vi "Dales Analog Read Pin.vi"(0 "Arduino Resource":T1={"VISA resource"="COM11", "Board Type"=enum."Uno", "Connection Type"=enum."USB / Serial", "Bytes Per Packet (15)"=15}, 7 "Analog Input Pin (0)":u8, 11 "error in":errorcluster) -> (4 "Arduino Resource":T1={"VISA resource"="COM11", "Board Type"=enum."Uno", "Connection Type"=enum."USB / Serial", "Bytes Per Packet (15)"=15}, 15 "error out":errorcluster)   [LabVIEW 2010]
doc: "Reads the analog voltage on the selected Arduino analog input pin (A0 - A5)."
uses:
  <vilib>/LabVIEW Interface for Arduino/Type Defs/Arduino Resource.ctl
  <vilib>/LabVIEW Interface for Arduino/Type Defs/Board Type.ctl
  <vilib>/LabVIEW Interface for Arduino/LabVIEW Interface for Arduino.lvlib
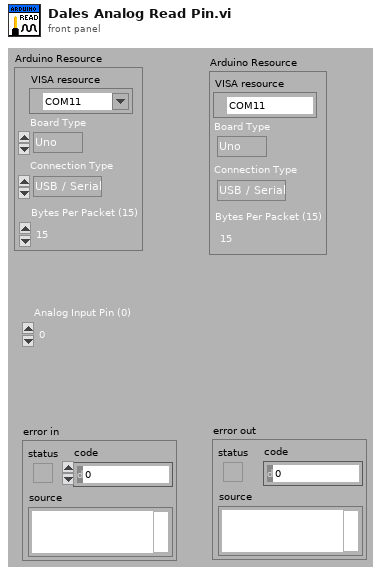
[diagram p1: front panel]
types:
  T1 = typedef "LabVIEW Interface for Arduino.lvlib/Arduino Resource.ctl" = cluster{"VISA resource":refnum<visa-resource-name>, "Board Type":T2, "Connection Type":enum8{"USB / Serial"}, "Bytes Per Packet (15)":u8}
  T2 = typedef "LabVIEW Interface for Arduino.lvlib/Board Type.ctl" = enum16{"Uno", "Dimuelanove w/Atmega 328", "Mega 2560"}
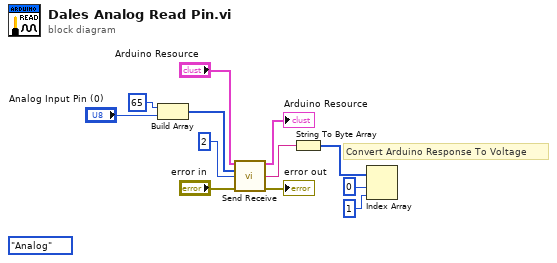
[diagram p0: block diagram]
diagram:
  (unwired) enum16{"Analog", "Digital"}."Analog" ("Pin Type")
  # "Convert Arduino Response To Voltage"
  n1 = Build Array(u8 65 ("element"), "Analog Input Pin (0)") -> (w9:u8[])
  n2 = call <vilib>:"Send Receive.vi"("Arduino Resource"="Arduino Resource", "Data"=w9, "Bytes To Read (0)"=u32 2, "error in"="error in") -> ("Arduino Resource"=→"Arduino Resource":T1, "Read Buffer"=w5:string, "error out"=→"error out":errorcluster)  [unwired: 9 in]
  n3 = String To Byte Array(string=w5) -> (unsigned byte array=w12:u8[])
  n4 = Index Array(array=w12, index #1=0 ("index"), index #2=1 ("index")) -> ()  [unwired: 2 out]
